vi "InitPerspective.vi"(4 "Far Clipping Plane":sgl, 6 "Near Clipping Plane":sgl, 8 "error in (no error)":errorcluster, 10 "Field of View":sgl, 11 "Control Window in":refnum<class "Control Window.lvclass">) -> (0 "error out":errorcluster, 3 "Control Window out":refnum<class "Control Window.lvclass">)   [LabVIEW 2015, in "Control Window.lvclass"]
uses:
  Control Window.lvclass
  Control Window.lvclass/Control Window.ctl
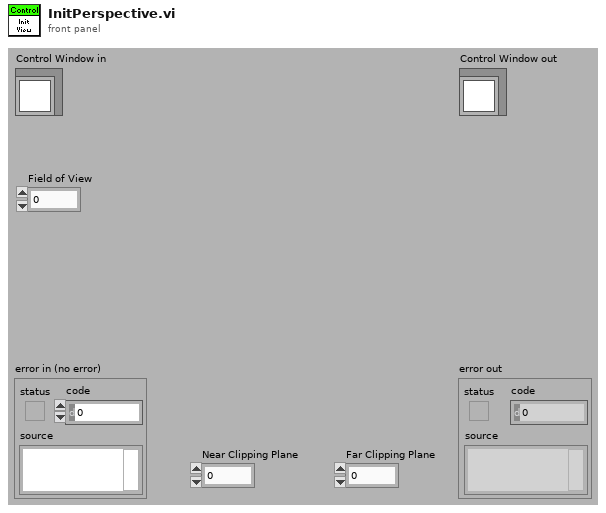
[diagram p1: front panel]
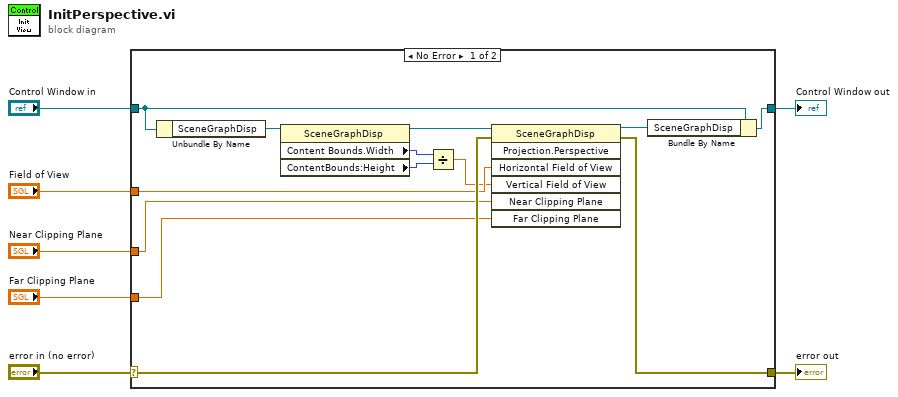
[diagram p0: block diagram]
diagram:
  n1 = case shown="No Error" "error in (no error)" {
    selector: "error in (no error)" -> [w17 w22]
    tunnel: [w16 w22] -> w6
    tunnel: [w19 w21] -> w4
    tunnel: "Control Window in" -> [w20 w21]
    tunnel: "Field of View" -> [w15 _]
    tunnel: "Near Clipping Plane" -> [w14 _]
    tunnel: "Far Clipping Plane" -> [w13 _]
    frame No Error {
      n2 = Unbundle By Name(w20) -> ("SceneGraphDisp"=w12:refnum<vi>)
      n3 = property class="SceneGraphDisp"(reference=w12) -> (reference out=w11:refnum<vi>, "Content Bounds.Width"=w10:u32, "ContentBounds:Height"=w9:u32)  [unwired: 1 in, 1 out]
      n4 = Divide(x=w10, y=w9) -> (x/y=w8:dbl)
      n5 = invoke class="SceneGraphDisp" method="Projection.Perspective"(reference=w11, error in=w17, "Horizontal Field of View"=w15, "Vertical Field of View"=w8, "Near Clipping Plane"=w14, "Far Clipping Plane"=w13) -> (reference out=w18:refnum<vi>, error out=w16:errorcluster)  [unwired: 1 in, 5 out]
      n6 = Bundle By Name(cluster=w20, "SceneGraphDisp"=w18) -> (w19:refnum<class "Control Window.lvclass">)
    }
    frame Error {
    }
  }
  "error out" <- w6
  "Control Window out" <- w4
